vi "MakeExample.vi"(8 "error in (no error)":errorcluster, 9 "TriggerRefractoryPeriod (Frames)":i32, 10 "StimulusObject Parameters":variant, 11 "TriggerOnTurnsTwoColors in":refnum<class "TriggerOnTurnsTwoColors.lvclass">) -> (0 "error out":errorcluster, 3 "TriggerOnTurnsTwoColors out":refnum<class "TriggerOnTurnsTwoColors.lvclass">)   [LabVIEW 2019, in "TriggerOnTurnsTwoColors.lvclass"]
uses:
  TriggerOnTurnsTwoColors.lvclass
  TriggerOnTurnsTwoColorsInputCluster.ctl
  TriggerOnTurnsTwoColors.lvclass/TriggerOnTurnsTwoColors.ctl
  ParametersGlobal.vi
  StimulusObject.lvclass
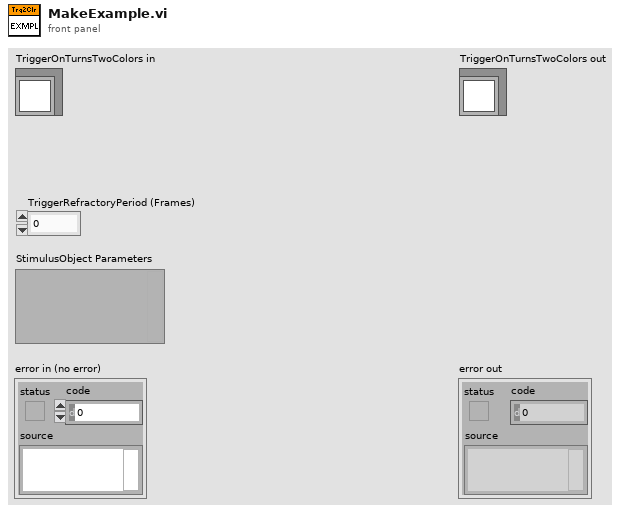
[diagram p1: front panel]
types:
  T1 = typedef "TriggerOnTurnsTwoColors.lvclass/TriggerOnTurnsTwoColorsInputCluster.ctl" = cluster{"Constant Intensity (uW/mm^2, negative is blue)":sgl, "dot radius (mm)":sgl, "BlueIntensity (uW/mm^2, negative is blue)":sgl[], "Durations (s)":sgl[], "Inter trigger interval (s)":dbl, "Ellipse Ratio Trigger Point":sgl, "RedIntensity (uW/mm^2, positive is red)":sgl[]}
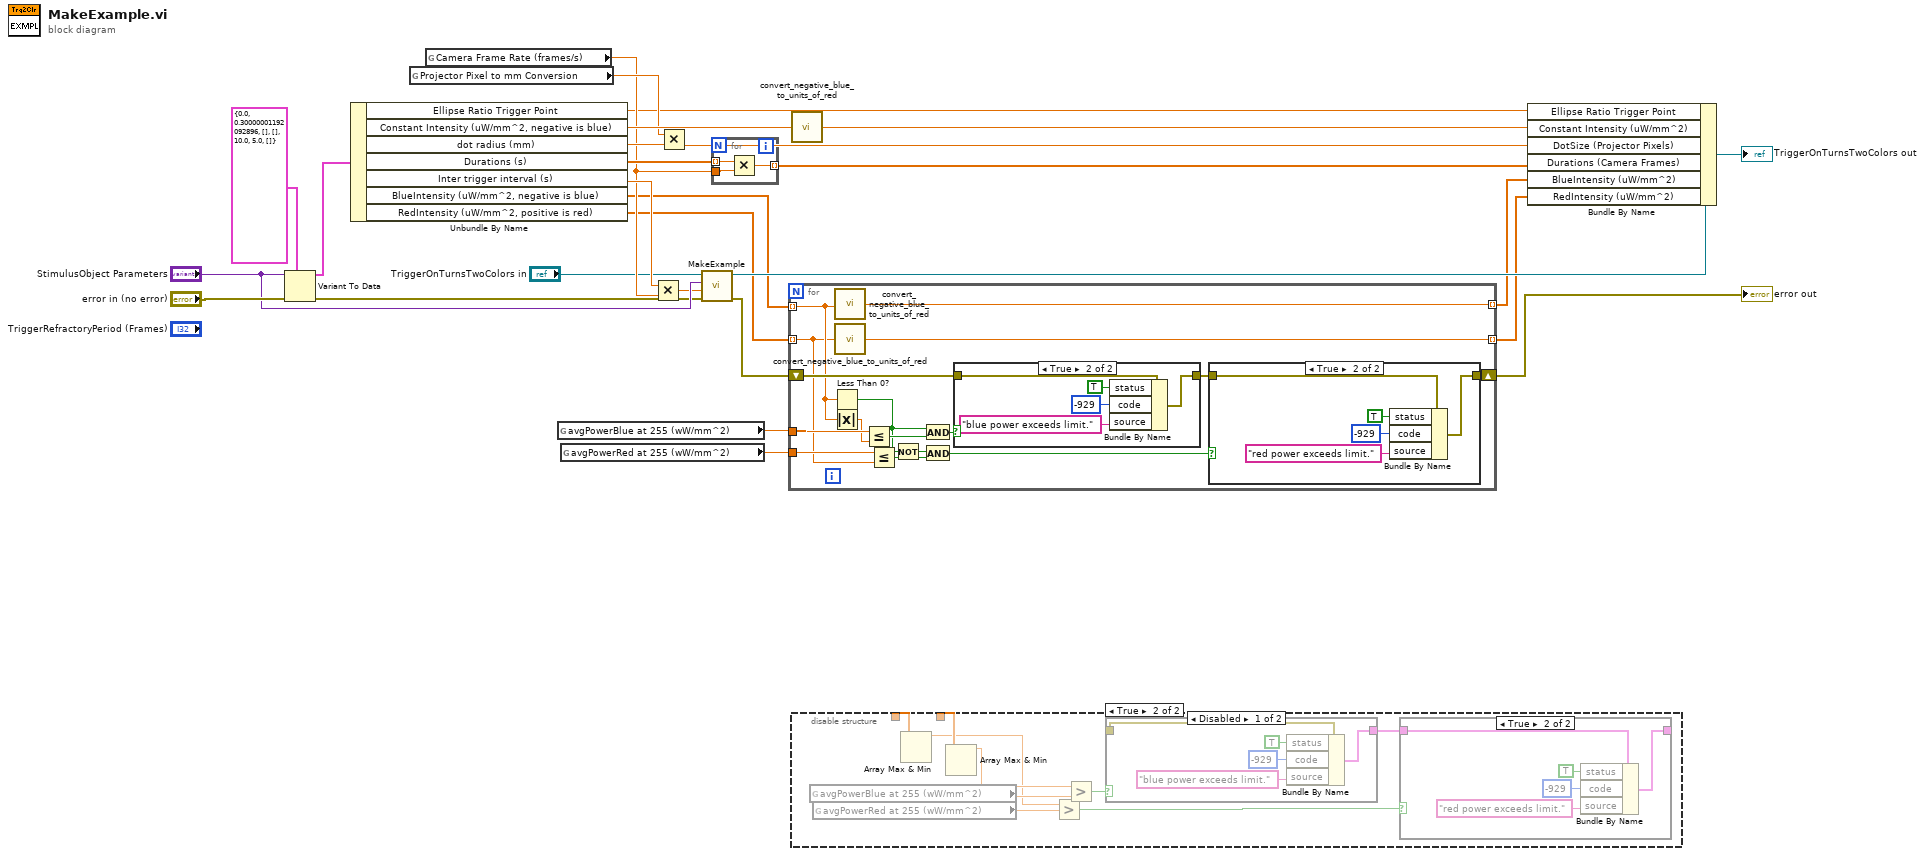
[diagram p0: block diagram]
diagram:
  n1 = Variant To Data(error in="error in (no error)", type=T1 {"Constant Intensity (uW/mm^2, negative is blue)"=0.0, "dot radius (mm)"=0.3, "BlueIntensity (uW/mm^2, negative is blue)"=[], "Durations (s)"=[], "Inter trigger interval (s)"=10.0, "Ellipse Ratio Trigger Point"=5.0, "RedIntensity (uW/mm^2, positive is red)"=[]} ("TriggerOnTurnsTwoColorsInputCluster"), Variant="StimulusObject Parameters") -> (data=w27:T1, error out=w11:errorcluster)
  n2 = Unbundle By Name(w27) -> ("Ellipse Ratio Trigger Point"=w17:sgl, "Constant Intensity (uW/mm^2, negative is blue)"=w25:sgl, "dot radius (mm)"=w23:sgl, "Durations (s)"=w20:sgl[], "Inter trigger interval (s)"=w26:dbl, "BlueIntensity (uW/mm^2, negative is blue)"=w4:sgl[], "RedIntensity (uW/mm^2, positive is red)"=w2:sgl[])
  n3 = global read "ParametersGlobal.vi" "Projector Pixel to mm Conversion"() -> (w22:sgl)
  n4 = global read "ParametersGlobal.vi" "Camera Frame Rate (frames/s)"() -> (w19:sgl)
  n5 = global read "ParametersGlobal.vi" "avgPowerBlue at 255 (wW/mm^2)"() -> (w6:sgl)
  n6 = global read "ParametersGlobal.vi" "avgPowerRed at 255 (wW/mm^2)"() -> (w5:sgl)
  n7 = Multiply(x=w26, y=w19) -> (x*y=w10:dbl)
  n8 = Multiply(x=w22, y=w23) -> (x*y=w21:sgl)
  n9 = call-parent "MakeExample.vi"("error in (no error)"=w11, "TriggerRefractoryPeriod (Frames)"=w10, "StimulusObject Parameters"="StimulusObject Parameters", "StimulusObject in"="TriggerOnTurnsTwoColors in") -> ("error out"=w7:errorcluster, "StimulusObject out"=w14:refnum<class "TriggerOnTurnsTwoColors.lvclass">)  [unwired: 6 in]
  n10 = for {
    tunnel: w20 -> [w30] mode=indexing
    tunnel: w19 -> [w29]
    tunnel: [w28] -> w18 mode=indexing
    n11 = Multiply(x=w30, y=w29) -> (x*y=w28:sgl)
  }
  n12 = for {
    tunnel: w4 -> [w33] mode=indexing
    shift-right: [w44] -> w8
    shift-left: w7 -> [w45]
    tunnel: w6 -> [w43]
    tunnel: w5 -> [w42]
    tunnel: [w41] -> w3 mode=indexing
    tunnel: w2 -> [w31] mode=indexing
    tunnel: [w32] -> w1 mode=indexing
    n13 = Less Than 0?(x=w33) -> (x < 0?=w34:bool)
    n14 = Absolute Value(x=w33) -> (abs(x)=w40:sgl)
    n15 = call "convert_negative_blue_to_units_of_red.vi"("Intensity in units of red (positive) and blue (negative)"=w33) -> ("Intensity in units of red (positive and negative)"=w41:sgl)
    n16 = call "convert_negative_blue_to_units_of_red.vi"("Intensity in units of red (positive) and blue (negative)"=w31) -> ("Intensity in units of red (positive and negative)"=w32:sgl)
    n17 = Less Or Equal?(x=w43, y=w40) -> (x <= y?=w39:bool)
    n18 = Less Or Equal?(x=w42, y=w31) -> (x <= y?=w36:bool)
    n19 = Not(x=w34) -> (.not. x?=w35:bool)
    n20 = And(x=w34, y=w39) -> (x .and. y?=w38:bool)
    n21 = And(x=w35, y=w36) -> (x .and. y?=w37:bool)
    n22 = case shown="True" w38 {
      tunnel: w45 -> [w53 w58]
      tunnel: [w53 w57] -> w46
      frame False {
      }
      frame True {
        n23 = Bundle By Name(cluster=w58, "status"=TRUE, "code"=-929, "source"="blue power exceeds limit.") -> (w57:errorcluster)
      }
    }
    n24 = case shown="True" w37 {
      tunnel: w46 -> [w47 w52]
      tunnel: [w47 w51] -> w44
      frame False {
      }
      frame True {
        n25 = Bundle By Name(cluster=w52, "status"=TRUE, "code"=-929, "source"="red power exceeds limit.") -> (w51:errorcluster)
      }
    }
  }
  "error out" <- w8
  n26 = call "convert_negative_blue_to_units_of_red.vi"("Intensity in units of red (positive) and blue (negative)"=w25) -> ("Intensity in units of red (positive and negative)"=w24:sgl)
  n27 = disable-structure shown="Disabled" {
    disable-tunnel: _ -> [w63 _]
    disable-tunnel: _ -> [w61 _]
    frame Disabled {
      n28 = global read "ParametersGlobal.vi" "avgPowerBlue at 255 (wW/mm^2)"() -> (w67:sgl)
      n29 = global read "ParametersGlobal.vi" "avgPowerRed at 255 (wW/mm^2)"() -> (w59:sgl)
      n30 = Array Max & Min(array=w61) -> (max value=w60:dbl)  [unwired: 3 out]
      n31 = Array Max & Min(array=w63) -> (max value=w62:dbl)  [unwired: 3 out]
      n32 = Greater?(x=w60, y=w59) -> (0:w64:bool)
      n33 = Greater?(x=w62, y=w67) -> (0:w66:bool)
      n34 = case shown="True" w66 {
        tunnel: _ -> [w74 w79]
        tunnel: [w74 w78] -> w65
        frame False {
        }
        frame True {
          n35 = Bundle By Name(cluster=w79, "status"=TRUE, "code"=-929, "source"="blue power exceeds limit.") -> (w78:cluster{})
        }
      }
      n36 = case shown="True" w64 {
        tunnel: w65 -> [w68 w73]
        tunnel: [w68 w72] -> _
        frame False {
        }
        frame True {
          n37 = Bundle By Name(cluster=w73, "status"=TRUE, "code"=-929, "source"="red power exceeds limit.") -> (w72:cluster{})
        }
      }
    }
    frame Enabled {
    }
  }
  n38 = Bundle By Name(cluster=w14, "Ellipse Ratio Trigger Point"=w17, "Constant Intensity (uW/mm^2)"=w24, "DotSize (Projector Pixels)"=w21, "Durations (Camera Frames)"=w18, "BlueIntensity (uW/mm^2)"=w3, "RedIntensity (uW/mm^2)"=w1) -> (→"TriggerOnTurnsTwoColors out":refnum<class "TriggerOnTurnsTwoColors.lvclass">)
